vi "UpdateData.vi"(1 "Duration Time (ms)":sgl, 4 "Detector Select":enum32{"4 Detectors", "8 Detectors"}(radio)=enum."8 Detectors", 5 "Delay Time":sgl[](array[numeric])) -> (0 "Elapsed Time(s)":sgl, 6 "Intensity Array":sgl[](array[numeric]), 7 "Tau Array":sgl[](array[numeric]), 8 "mean":dbl format="%0.2f", 9 "mean 8":dbl format="%0.2f", 10 "mean 2":dbl format="%0.2f", 11 "mean 7":dbl format="%0.2f", 12 "mean 3":dbl format="%0.2f", 13 "Intensity data":string, 14 "g2 Display":cluster{"Delay Time":sgl[], sgl[]}[](array[cluster]), 15 "mean 4":dbl format="%0.2f", 16 "mean 5":dbl format="%0.2f", 17 "mean 6":dbl format="%0.2f", 18 "tau data":string, 19 "g2 data":string)   [LabVIEW 2016]
uses:
  GTcode_v6_Michelle/flex05-4chPascal.dll
  GTcode_v6_Michelle/flex05oem8chauto100nsPASCAL_win7.dll
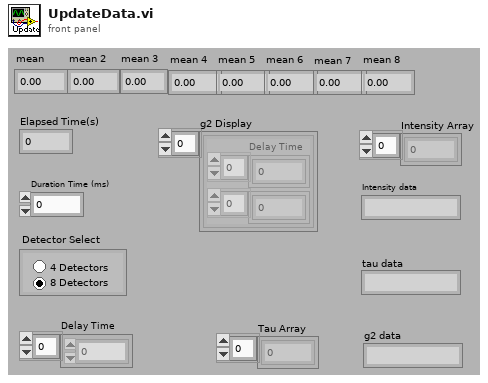
[diagram p1: front panel]
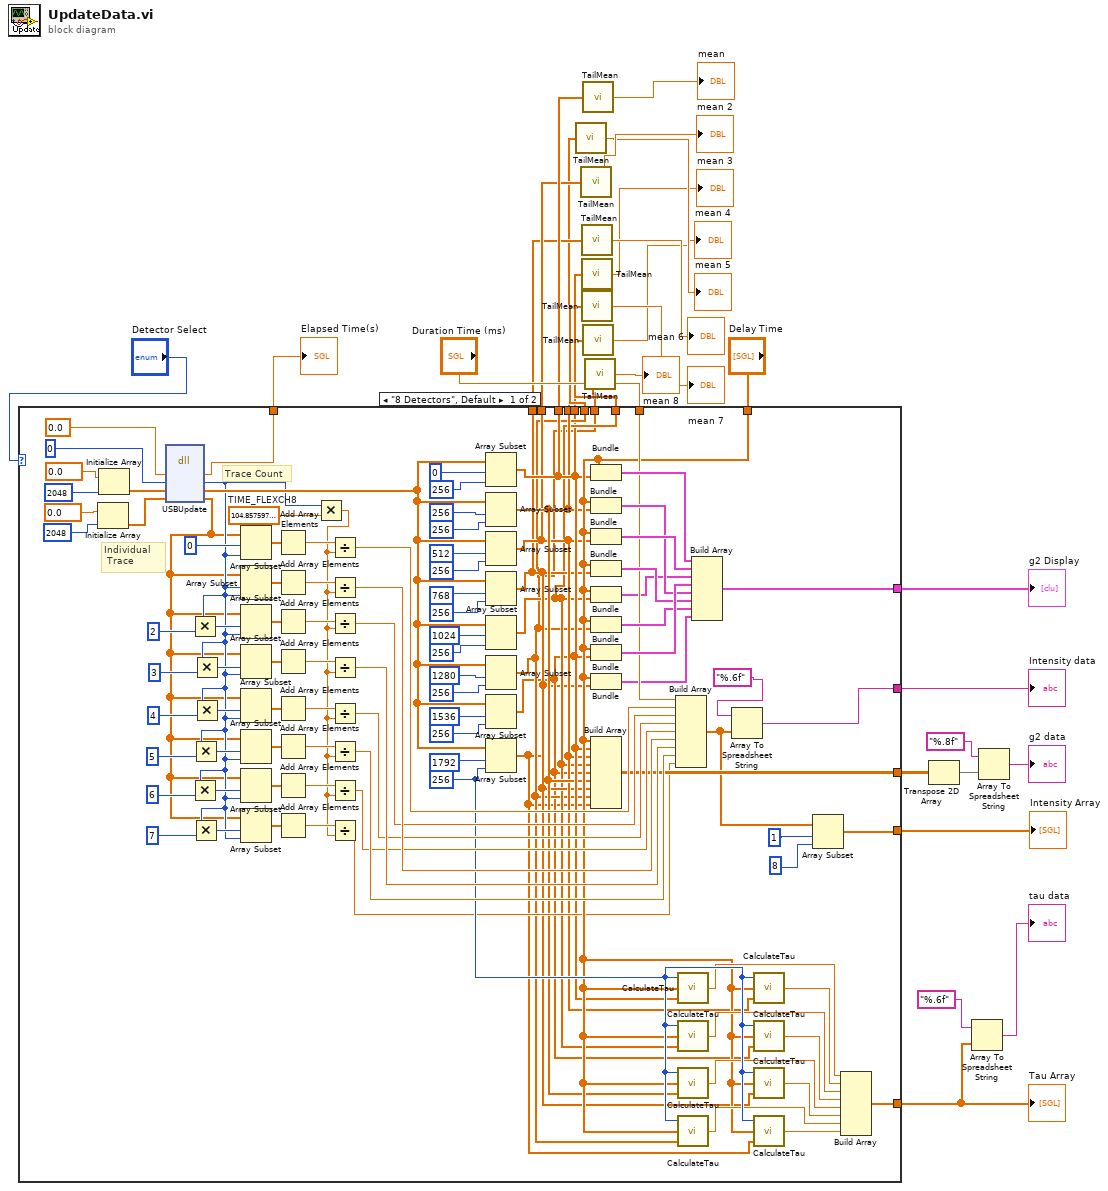
[diagram p0: block diagram]
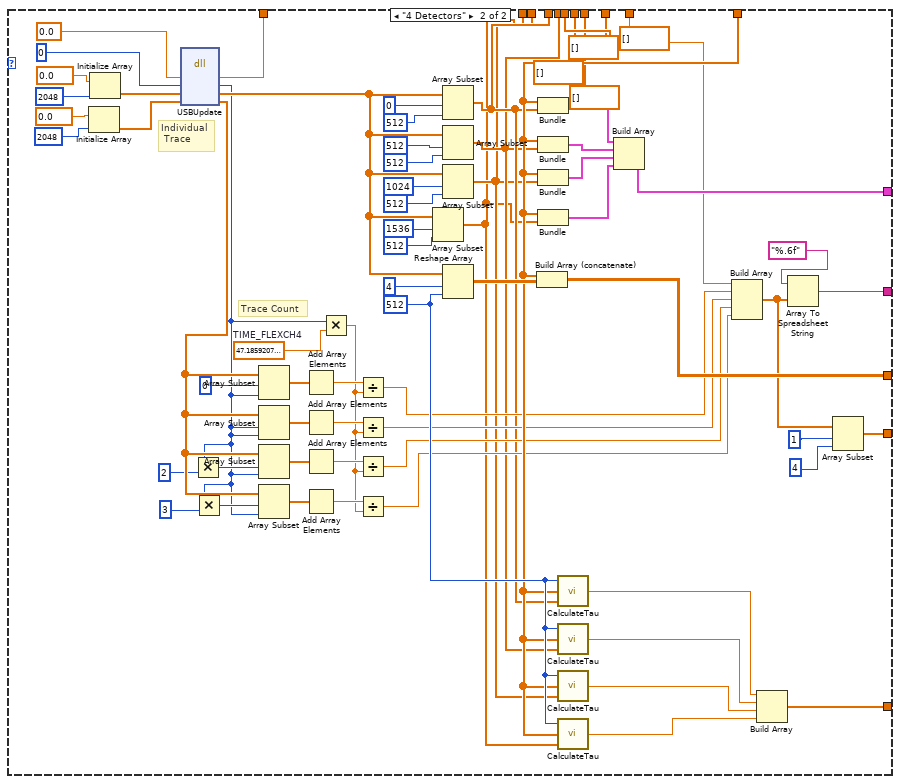
[diagram p2: hidden frame]
diagram:
  n1 = case shown="\"8 Detectors\", Default" "Detector Select" {
    tunnel: [w56 w188] -> w25
    tunnel: [w116 w187] -> w27
    tunnel: [w66 w185] -> w20
    tunnel: "Duration Time (ms)" -> [w77 w141]
    tunnel: [w69 w166] -> w26
    tunnel: "Delay Time" -> [w54 w160]
    tunnel: [w53 w159] -> w23
    tunnel: [w49 w143] -> w30
    tunnel: [w38 w140] -> w16
    tunnel: [w37 w139] -> w7
    tunnel: [w36 w138] -> w13
    tunnel: [w35 w137] -> w12
    tunnel: [w34 sgl[] []] -> w11
    tunnel: [w33 sgl[] []] -> w10
    tunnel: [w32 sgl[] []] -> w9
    tunnel: [w31 sgl[] []] -> w8
    frame "8 Detectors", Default {
      w106 = sgl 104.8576  # TIME_FLEXCH8
      w65 = 256
      # "Individual\n Trace"
      # "Trace Count"
      n2 = Initialize Array(sgl 0.0 ("Element Data"), 2048 ("Dimension Size")) -> (w42:sgl[])
      n3 = Initialize Array(sgl 0.0 ("Element Data"), 2048 ("Dimension Size")) -> (w43:sgl[])
      n4 = dll-call lib="C:/Users/BUCKLEY-ADMIN/Desktop/GTcode_v6_Michelle/flex05oem8chauto100nsPASCAL_win7.dll" fn="USBUpdate" label="UpdateCH8"("arg1"=sgl 0.0 ("Input Value"), "arg2"=u16 0 ("Input Value"), "arg3"=w43, "arg4"=w42) -> ("arg1"=w56:sgl, "arg2"=w78:u16, "arg3"=w96:sgl[], "arg4"=w55:sgl[])  [unwired: 4 in, 2 out]
      n5 = Multiply(x=w78, y=2) -> (x*y=w90:i32)
      n6 = Multiply(x=w78, y=6) -> (x*y=w87:i32)
      n7 = Multiply(x=w78, y=5) -> (x*y=w88:i32)
      n8 = Multiply(x=w78, y=7) -> (x*y=w86:i32)
      n9 = Multiply(x=w78, y=3) -> (x*y=w85:i32)
      n10 = Multiply(x=w78, y=4) -> (x*y=w89:i32)
      n11 = Array Subset(array=w55, index=0, length=w78) -> (w114:sgl[])
      n12 = Array Subset(array=w55, index=w78, length=w78) -> (w113:sgl[])
      n13 = Array Subset(array=w55, index=w90, length=w78) -> (w112:sgl[])
      n14 = Array Subset(array=w55, index=w85, length=w78) -> (w111:sgl[])
      n15 = Array Subset(array=w55, index=w89, length=w78) -> (w110:sgl[])
      n16 = Array Subset(array=w55, index=w88, length=w78) -> (w109:sgl[])
      n17 = Array Subset(array=w55, index=w87, length=w78) -> (w108:sgl[])
      n18 = Array Subset(array=w55, index=w86, length=w78) -> (w107:sgl[])
      n19 = Add Array Elements(numeric array=w114) -> (sum=w105:sgl)
      n20 = Add Array Elements(numeric array=w113) -> (sum=w104:sgl)
      n21 = Add Array Elements(numeric array=w112) -> (sum=w103:sgl)
      n22 = Add Array Elements(numeric array=w111) -> (sum=w102:sgl)
      n23 = Add Array Elements(numeric array=w110) -> (sum=w101:sgl)
      n24 = Add Array Elements(numeric array=w109) -> (sum=w100:sgl)
      n25 = Add Array Elements(numeric array=w108) -> (sum=w99:sgl)
      n26 = Add Array Elements(numeric array=w107) -> (sum=w98:sgl)
      n27 = Multiply(x=w78, y=w106) -> (x*y=w97:sgl)
      n28 = Divide(x=w105, y=w97) -> (x/y=w70:sgl)
      n29 = Divide(x=w104, y=w97) -> (x/y=w74:sgl)
      n30 = Divide(x=w103, y=w97) -> (x/y=w71:sgl)
      n31 = Divide(x=w102, y=w97) -> (x/y=w75:sgl)
      n32 = Divide(x=w101, y=w97) -> (x/y=w72:sgl)
      n33 = Divide(x=w100, y=w97) -> (x/y=w76:sgl)
      n34 = Divide(x=w99, y=w97) -> (x/y=w73:sgl)
      n35 = Divide(x=w98, y=w97) -> (x/y=w40:sgl)
      n36 = Array Subset(array=w96, index=0, length=256) -> (w38:sgl[])
      n37 = Array Subset(array=w96, index=256, length=256) -> (w37:sgl[])
      n38 = Array Subset(array=w96, index=512, length=256) -> (w36:sgl[])
      n39 = Array Subset(array=w96, index=768, length=256) -> (w35:sgl[])
      n40 = Array Subset(array=w96, index=1024, length=256) -> (w34:sgl[])
      n41 = Array Subset(array=w96, index=1280, length=256) -> (w33:sgl[])
      n42 = Array Subset(array=w96, index=1536, length=256) -> (w32:sgl[])
      n43 = Array Subset(array=w96, index=1792, length=w65) -> (w31:sgl[])
      n44 = Bundle("Delay Time"=w54, w38) -> (w124:cluster{"Delay Time":sgl[], sgl[]})  [unwired: 1 in]
      n45 = Bundle("Delay Time"=w54, w37) -> (w93:cluster{"Delay Time":sgl[], sgl[]})  [unwired: 1 in]
      n46 = Bundle("Delay Time"=w54, w36) -> (w95:cluster{"Delay Time":sgl[], sgl[]})  [unwired: 1 in]
      n47 = Bundle("Delay Time"=w54, w35) -> (w92:cluster{"Delay Time":sgl[], sgl[]})  [unwired: 1 in]
      n48 = Bundle("Delay Time"=w54, w34) -> (w67:cluster{"Delay Time":sgl[], sgl[]})  [unwired: 1 in]
      n49 = Bundle("Delay Time"=w54, w33) -> (w91:cluster{"Delay Time":sgl[], sgl[]})  [unwired: 1 in]
      n50 = Bundle("Delay Time"=w54, w32) -> (w94:cluster{"Delay Time":sgl[], sgl[]})  [unwired: 1 in]
      n51 = Bundle("Delay Time"=w54, w31) -> (w68:cluster{"Delay Time":sgl[], sgl[]})  [unwired: 1 in]
      n52 = Build Array(w54, w38, w36, w34, w32, w37, w35, w33, w31) -> (w66:sgl[][])
      n53 = Build Array(w77, w70, w71, w72, w73, w74, w75, w76, w40) -> (w39:sgl[])
      n54 = call "CalculateTau.vi"("g2 data"=w38, "delaytime"=w54, "array size"=w65) -> ("Tau"=w64:sgl)
      n55 = call "CalculateTau.vi"("g2 data"=w34, "delaytime"=w54, "array size"=w65) -> ("Tau"=w62:sgl)
      n56 = call "CalculateTau.vi"("g2 data"=w37, "delaytime"=w54, "array size"=w65) -> ("Tau"=w60:sgl)
      n57 = call "CalculateTau.vi"("g2 data"=w33, "delaytime"=w54, "array size"=w65) -> ("Tau"=w58:sgl)
      n58 = Build Array(w124, w95, w67, w94, w93, w92, w91, w68) -> (w116:cluster{"Delay Time":sgl[], sgl[]}[])
      n59 = Array To Spreadsheet String(array=w39, 3:"%.6f") -> (spreadsheet string=w69:string)  [unwired: 1 in]
      n60 = call "CalculateTau.vi"("g2 data"=w36, "delaytime"=w54, "array size"=w65) -> ("Tau"=w63:sgl)
      n61 = call "CalculateTau.vi"("g2 data"=w32, "delaytime"=w54, "array size"=w65) -> ("Tau"=w61:sgl)
      n62 = call "CalculateTau.vi"("g2 data"=w35, "delaytime"=w54, "array size"=w65) -> ("Tau"=w59:sgl)
      n63 = call "CalculateTau.vi"("g2 data"=w31, "delaytime"=w54, "array size"=w65) -> ("Tau"=w57:sgl)
      n64 = Array Subset(array=w39, index=1, length=8) -> (w49:sgl[])
      n65 = Build Array(w64, w63, w62, w61, w60, w59, w58, w57) -> (w53:sgl[])
    }
    frame "4 Detectors" {
      w182 = sgl 47.18592  # TIME_FLEXCH4
      w165 = 512
      # "Individual\n Trace"
      # "Trace Count"
      n66 = Initialize Array(sgl 0.0 ("Element Data"), 2048 ("Dimension Size")) -> (w146:sgl[])
      n67 = Initialize Array(sgl 0.0 ("Element Data"), 2048 ("Dimension Size")) -> (w147:sgl[])
      n68 = dll-call lib="C:/Users/BUCKLEY-ADMIN/Desktop/GTcode_v6_Michelle/flex05-4chPascal.dll" fn="USBUpdate" label="UpdateCH4"(sgl 0.0 ("Input Value"), u16 0 ("Input Value"), w147, "arg4"=w146) -> (w188:sgl, w167:u16, w172:sgl[], "arg4"=w183:sgl[])  [unwired: 4 in, 2 out]
      n69 = Multiply(x=w167, y=2) -> (x*y=w170:i32)
      n70 = Multiply(x=w167, y=3) -> (x*y=w168:i32)
      n71 = Array Subset(array=w183, index=0, length=w167) -> (w177:sgl[])
      n72 = Array Subset(array=w183, index=w167, length=w167) -> (w176:sgl[])
      n73 = Array Subset(array=w183, index=w170, length=w167) -> (w175:sgl[])
      n74 = Array Subset(array=w183, index=w168, length=w167) -> (w174:sgl[])
      n75 = Add Array Elements(numeric array=w177) -> (sum=w181:sgl)
      n76 = Add Array Elements(numeric array=w176) -> (sum=w180:sgl)
      n77 = Add Array Elements(numeric array=w175) -> (sum=w179:sgl)
      n78 = Add Array Elements(numeric array=w174) -> (sum=w178:sgl)
      n79 = Multiply(x=w167, y=w182) -> (x*y=w173:sgl)
      n80 = Divide(x=w181, y=w173) -> (x/y=w158:sgl)
      n81 = Divide(x=w180, y=w173) -> (x/y=w157:sgl)
      n82 = Divide(x=w179, y=w173) -> (x/y=w156:sgl)
      n83 = Divide(x=w178, y=w173) -> (x/y=w155:sgl)
      n84 = Array Subset(array=w172, index=1536, length=512) -> (w137:sgl[])
      n85 = Array Subset(array=w172, index=0, length=512) -> (w140:sgl[])
      n86 = Array Subset(array=w172, index=512, length=512) -> (w139:sgl[])
      n87 = Array Subset(array=w172, index=1024, length=512) -> (w138:sgl[])
      n88 = Reshape Array(w172, 4, w165) -> (w186:sgl[][])
      n89 = Build Array (concatenate)(w160, w186) -> (w185:sgl[][])
      n90 = Bundle("Delay Time"=w160, w140) -> (w192:cluster{"Delay Time":sgl[], sgl[]})  [unwired: 1 in]
      n91 = Bundle("Delay Time"=w160, w139) -> (w191:cluster{"Delay Time":sgl[], sgl[]})  [unwired: 1 in]
      n92 = Bundle("Delay Time"=w160, w138) -> (w190:cluster{"Delay Time":sgl[], sgl[]})  [unwired: 1 in]
      n93 = Bundle("Delay Time"=w160, w137) -> (w189:cluster{"Delay Time":sgl[], sgl[]})  [unwired: 1 in]
      n94 = call "CalculateTau.vi"("g2 data"=w140, "delaytime"=w160, "array size"=w165) -> ("Tau"=w164:sgl)
      n95 = call "CalculateTau.vi"("g2 data"=w139, "delaytime"=w160, "array size"=w165) -> ("Tau"=w163:sgl)
      n96 = call "CalculateTau.vi"("g2 data"=w138, "delaytime"=w160, "array size"=w165) -> ("Tau"=w162:sgl)
      n97 = call "CalculateTau.vi"("g2 data"=w137, "delaytime"=w160, "array size"=w165) -> ("Tau"=w161:sgl)
      n98 = Build Array(w192, w191, w190, w189) -> (w187:cluster{"Delay Time":sgl[], sgl[]}[])
      n99 = Build Array(w141, w158, w157, w156, w155) -> (w142:sgl[])
      n100 = Build Array(w164, w163, w162, w161) -> (w159:sgl[])
      n101 = Array To Spreadsheet String(array=w142, 3:"%.6f") -> (spreadsheet string=w166:string)  [unwired: 1 in]
      n102 = Array Subset(array=w142, index=1, length=4) -> (w143:sgl[])
    }
  }
  "Intensity Array" <- w30
  "Tau Array" <- w23
  "g2 Display" <- w27
  "Intensity data" <- w26
  "Elapsed Time(s)" <- w25
  n103 = call "TailMean.vi"("array"=w7) -> ("mean"=→"mean 5":dbl)
  n104 = call "TailMean.vi"("array"=w13) -> ("mean"=→"mean 2":dbl)
  n105 = call "TailMean.vi"("array"=w12) -> ("mean"=→"mean 6":dbl)
  n106 = call "TailMean.vi"("array"=w11) -> ("mean"=→"mean 3":dbl)
  n107 = call "TailMean.vi"("array"=w10) -> ("mean"=→"mean 7":dbl)
  n108 = call "TailMean.vi"("array"=w16) -> ("mean"=→"mean":dbl)
  n109 = call "TailMean.vi"("array"=w9) -> ("mean"=→"mean 4":dbl)
  n110 = call "TailMean.vi"("array"=w8) -> ("mean"=→"mean 8":dbl)
  n111 = Transpose 2D Array(2D array=w20) -> (transposed array=w21:sgl[][])
  n112 = Array To Spreadsheet String(array=w23, 3:"%.6f") -> (spreadsheet string=→"tau data":string)  [unwired: 1 in]
  n113 = Array To Spreadsheet String(array=w21, 3:"%.8f") -> (spreadsheet string=→"g2 data":string)  [unwired: 1 in]
